vi "Periodic Tasks.vi"(8 "error in":errorcluster) -> ()   [LabVIEW 2015]
doc: "This VI runs in parallel to other tasks. It can contain as many user-defined periodic loops as you need. These can carry out PID or other sorts of timed response."
uses:
  <vilib>/Rock Robotics/WPI/Solenoid/WPI_SolenoidValue.ctl
  <vilib>/Rock Robotics/WPI/Solenoid/WPI_SolenoidSetEnum.vi
  Robot Global Data.vi
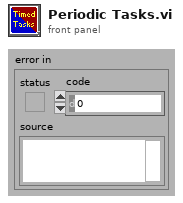
[diagram p1: front panel]
types:
  T1 = typedef "WPI_SolenoidValue.ctl" = enum16{"Off", "On", "Forward", "Reverse"}
  T2 = typedef "WPI_SolenoidDevRef.ctl" = cluster{"DevStatus":errorcluster, "Pneumatics Control Module":u8, "Forward Solenoid Channel":T3, "Reverse Solenoid Channel":T3}
  T3 = typedef "WPI_SolenoidChannel.ctl" = enum8{"Solenoid 0", "Solenoid 1", "Solenoid 2", "Solenoid 3", "Solenoid 4", "Solenoid 5", "Solenoid 6", "Solenoid 7", "Invalid"}
  T4 = typedef "WPI_MotorControlDeviceRef.ctl" = cluster{"DeviceStatus":errorcluster, "Type":T5, "PWM":cluster{"PWM Channel":T6, "DeadBand":T7}, "CAN":cluster{"Device Number":u8, "Control Mode":T8, "Semaphore":T9, "Max Vout":dbl, "TalonSRX Control Mode":T10}, "Invert":bool}
  T5 = typedef "WPI_MotorControlType.ctl" = enum16{"PWM", "CAN", "CANTalonSRX"}
  T6 = typedef "FPGA_DIOPWMChannel.ctl" = enum8{"PWM 0", "PWM 1", "PWM 2", "PWM 3", "PWM 4", "PWM 5", "PWM 6", "PWM 7", "PWM 8", "PWM 9", "PWM MXP 0", "PWM MXP 1", "PWM MXP 2", "PWM MXP 3", "PWM MXP 4", "PWM MXP 5", "PWM MXP 6", "PWM MXP 7", "PWM MXP 8", "PWM MXP 9", "Invalid"}
  T7 = typedef "WPI_PWMDeadband.ctl" = cluster{"Name":string, "maxPositivePwm":i32, "minPositivePwm":i32, "centerPwm":i32, "maxNegativePwm":i32, "minNegativePwm":i32, "angularRange":u16}
  T8 = typedef "WPI_CANJaguar_ControlMode.ctl" = enum8{"Percent VBus", "Current", "Speed", "Position", "Voltage"}
  T9 = typedef "Semaphore RefNum" = refnum<k1>
  T10 = typedef "WPI_CANTalonSRX_APIControlMode.ctl" = enum8{"Percent VBus", "Speed", "Position", "Slave", "Unchanged / Invalid", "Voltage Compensation", "Current", "Motion Profile"}
  T11 = typedef "WPI_PotentiometerDevRef.ctl" = cluster{"DevStatus":errorcluster, "Analog Channel":T12, "Invert Output":bool}
  T12 = typedef "FPGA_AIChannel.ctl" = enum8{"AI 0", "AI 1", "AI 2", "AI 3", "AI MXP 0", "AI MXP 1", "AI MXP 2", "AI MXP 3", "Invalid"}
  T13 = typedef "WPI_EncoderDevRef.ctl" = cluster{"DevStatus":errorcluster, "EncoderIndex":T14, "CounterIndex":T15, "DistancePerCount":dbl, "Decoding Type":T16}
  T14 = typedef "FPGA_EncoderIdx.ctl" = enum8{"Enc 0", "Enc 1", "Enc 2", "Enc 3", "Enc 4", "Enc 5", "Enc 6", "Enc 7", "Invalid"}
  T15 = typedef "FPGA_CounterCtrSystemIndex.ctl" = enum8{"Ctr 0", "Ctr 1", "Ctr 2", "Ctr 3", "Ctr 4", "Ctr 5", "Ctr 6", "Ctr 7", "Invalid"}
  T16 = typedef "WPI_EncoderType.ctl" = enum16{"1x", "2x", "4x"}
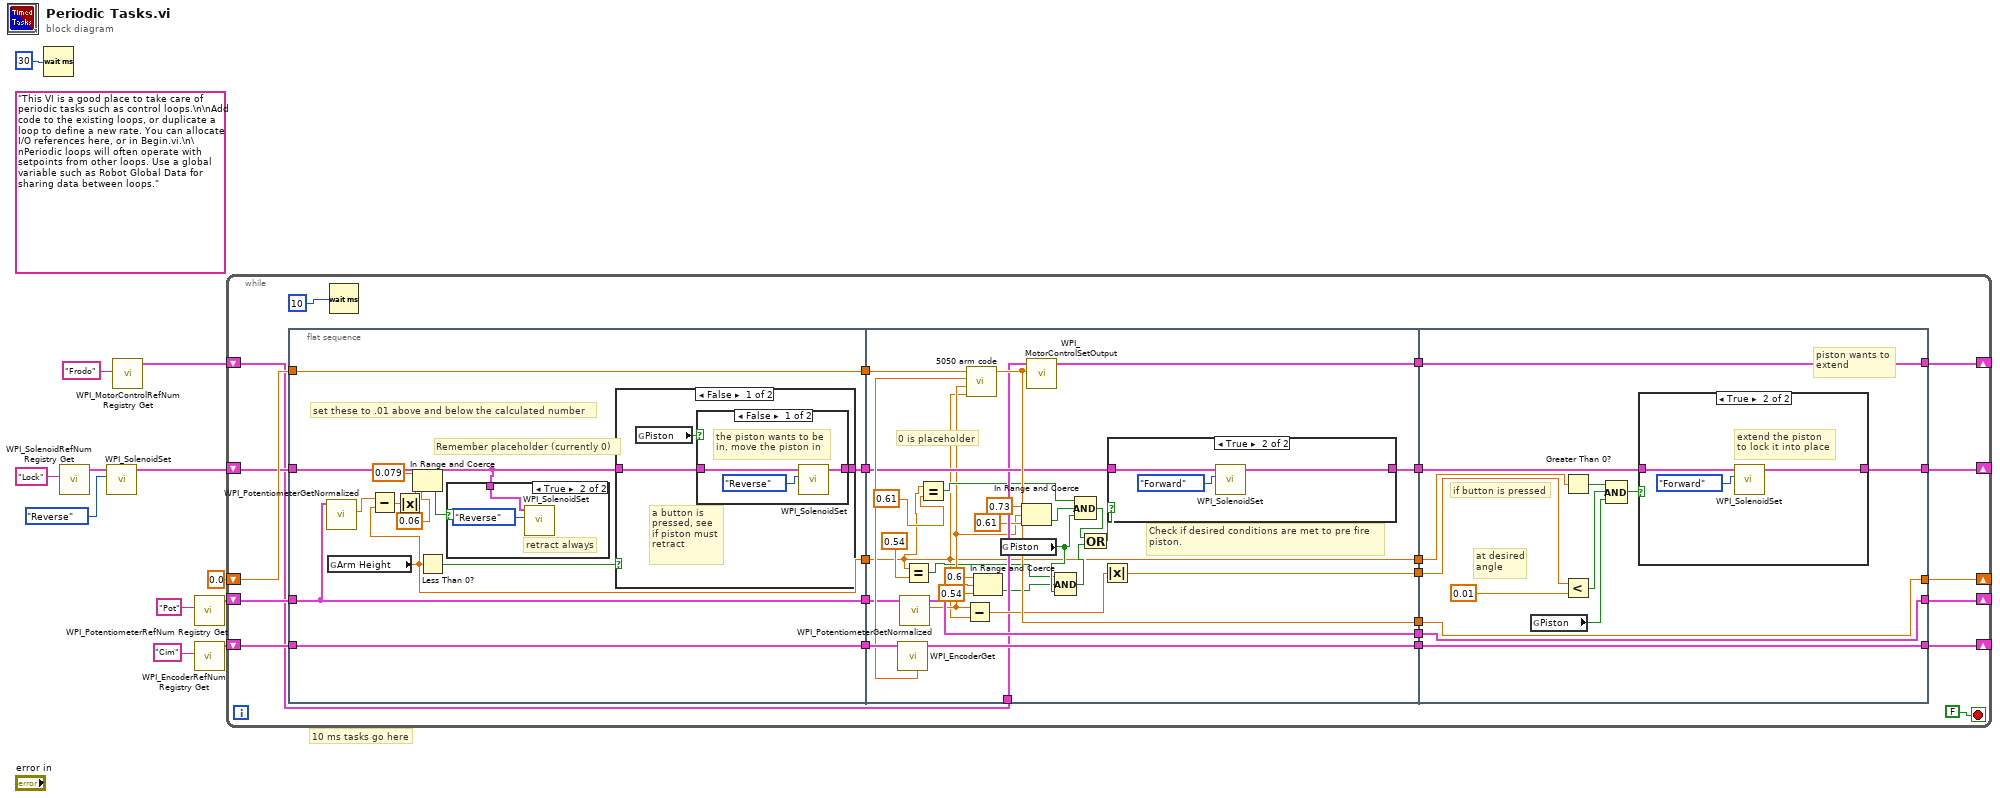
[diagram p0: block diagram]
diagram:
  (unwired) "This VI is a good place to take care of periodic tasks such as control loops.\n\nAdd code to the existing loops, or duplicate a loop to define a new rate. You can allocate I/O references here, or in Begin.vi.\n\nPeriodic loops will often operate with setpoints from other loops. Use a global variable such as Robot Global Data for sharing data between loops."
  # "10 ms tasks go here"
  n1 = Wait (ms)(milliseconds to wait=u32 30) -> ()  [unwired: 1 out]
  n2 = call <vilib>:"WPI_SolenoidRefNum Registry Get.vi"("refnum name"="Lock") -> ("SolenoidDevRef"=w4:T2)  [unwired: 9 in, 1 out]
  n3 = call-poly <vilib>:"WPI_SolenoidSet.vi"("Value"=WPI_SolenoidValue."Reverse", "SolenoidDevRef"=w4) -> ("SolenoidDevRef"=w3:T2)  [unwired: 8 in, 1 out]
  n4 = call <vilib>:"WPI_MotorControlRefNum Registry Get.vi"("refnum name"="Frodo") -> ("MotorControlDevRef"=w11:T4)  [unwired: 9 in, 1 out]
  n5 = call <vilib>:"WPI_PotentiometerRefNum Registry Get.vi"("refnum name"="Pot") -> ("PotDevRef"=w9:T11)  [unwired: 9 in, 1 out]
  n6 = call <vilib>:"WPI_EncoderRefNum Registry Get.vi"("refnum name"="Cim") -> ("EncoderDevRef"=w10:T13)  [unwired: 9 in, 1 out]
  n7 = while {
    shift-right: [w20] -> _
    shift-left: w11 -> [w14]
    shift-right: [w18] -> _
    shift-left: w9 -> [w15]
    shift-right: [w17] -> _
    shift-left: w10 -> [w22]
    shift-right: [w19] -> _
    shift-left: 0.0 -> [w24]
    shift-right: [w21] -> _
    shift-left: w3 -> [w23]
    stop <- FALSE stop-if-true
    n8 = flat-sequence {
      tunnel: w24 -> [w46]
      tunnel: w22 -> [w49]
      tunnel: [w49] -> w35
      tunnel: [w43] -> w34
      tunnel: w23 -> [w41]
      tunnel: [w47] -> w33
      tunnel: [w46] -> w32
      tunnel: [w45] -> w16
      tunnel: w15 -> [w45]
      tunnel: [w86] -> w31
      tunnel: [w85] -> w30
      tunnel: [w84] -> w29
      tunnel: [w83] -> w28
      tunnel: w35 -> [w88]
      tunnel: w34 -> [w60]
      tunnel: w33 -> [w80]
      tunnel: [w79] -> w27
      tunnel: [w60] -> w26
      tunnel: [w81] -> w25
      tunnel: w32 -> [w78]
      tunnel: w16 -> [w77]
      tunnel: w14 -> [w76]
      tunnel: [w102] -> w19
      tunnel: [w103] -> w18
      tunnel: [w104] -> w17
      tunnel: [w105] -> w20
      tunnel: w31 -> [w105]
      tunnel: w30 -> [w104]
      tunnel: w29 -> [w103]
      tunnel: w28 -> [w102]
      tunnel: w27 -> [w95]
      tunnel: w26 -> [w101]
      tunnel: w25 -> [w100]
      tunnel: [w94] -> w21
      frame #0 {
        # "set these to .01 above and below the calculated number"
        # "Remember placeholder (currently 0)"
        n9 = call <vilib>:"WPI_PotentiometerGetNormalized.vi"("PotDevRef"=w45) -> ("Normalized Value"=w44:dbl)  [unwired: 8 in, 2 out]
        n10 = global read "Robot Global Data.vi" "Arm Height"() -> (w43:dbl)
        n11 = Subtract(x=w44, y=w43) -> (x-y=w42:dbl)
        n12 = Absolute Value(x=w42) -> (abs(x)=w40:dbl)
        n13 = In Range and Coerce(upper limit=0.079, x=w40, lower limit=0.06 ("y")) -> (In Range?=w37:bool)  [unwired: 1 out]
        n14 = Less Than 0?(x=w43) -> (x < 0?=w48:bool)
        n15 = case shown="True" w37 {
          tunnel: w41 -> [_ w50]
          frame False {
            # "do nothing?"
          }
          frame True {
            # "retract always"
            n16 = call-poly <vilib>:"WPI_SolenoidSet.vi"("Value"=WPI_SolenoidValue."Reverse", "SolenoidDevRef"=w50) -> ()  [unwired: 8 in, 2 out]
          }
        }
        n17 = case shown="False" w48 {
          tunnel: w41 -> [w53 w59]
          tunnel: [w54 w59] -> w47
          frame False {
            # "a button is\npressed, see\nif piston must\nretract"
            n18 = global read "Robot Global Data.vi" "Piston"() -> (w52:bool)
            n19 = case shown="False" w52 {
              tunnel: [w55 w58] -> w54
              tunnel: w53 -> [w57 w58]
              frame False {
                # "the piston wants to be\nin, move the piston in"
                n20 = call-poly <vilib>:"WPI_SolenoidSet.vi"("Value"=WPI_SolenoidValue."Reverse", "SolenoidDevRef"=w57) -> ("SolenoidDevRef"=w55:T2)  [unwired: 8 in, 1 out]
              }
              frame True {
                # "the piston wants to\nbe out, do not extend\npiston yet"
              }
            }
          }
          frame True {
            # "no button is pressed\ndo not change piston position"
          }
        }
      }
      frame #1 {
        # "0 is placeholder"
        # "Check if desired conditions are met to pre fire piston."
        n21 = call <vilib>:"WPI_EncoderGet.vi"("EncoderDevRef"=w88) -> ("EncoderDevRef"=w85:T13, "Rate"=w87:dbl)  [unwired: 5 in, 4 out]
        n22 = call <vilib>:"WPI_PotentiometerGetNormalized.vi"("PotDevRef"=w77) -> ("Normalized Value"=w65:dbl, "PotDevRef"=w84:T11)  [unwired: 8 in, 1 out]
        n23 = Equal?(x=w60, y=0.54) -> (x = y?=w62:bool)
        n24 = Equal?(x=w60, y=0.61 ("value")) -> (x = y?=w71:bool)
        n25 = Subtract(x=w65, y=w60) -> (x-y=w82:dbl)
        n26 = call "5050 arm code.vi"("desiredAngle"=w60, "potAngle"=w65, "encoderHz"=w87, "initSpeed"=w78) -> ("motorSpeed"=w83:dbl)  [unwired: 7 in]
        n27 = In Range and Coerce(upper limit=0.6, x=w65, lower limit=0.54) -> (In Range?=w66:bool)  [unwired: 1 out]
        n28 = global read "Robot Global Data.vi" "Piston"() -> (w67:bool)
        n29 = In Range and Coerce(upper limit=0.73, x=w65, lower limit=0.61) -> (In Range?=w72:bool)  [unwired: 1 out]
        n30 = call <vilib>:"WPI_MotorControlSetOutput.vi"("Output"=w83, "MotorControlDevRef"=w76) -> ("MotorControlDevRef"=w86:T4)  [unwired: 7 in, 2 out]
        n31 = Compound Arithmetic op=AND(w62, w66, w67) -> (w68:bool)
        n32 = Compound Arithmetic op=AND(w71, w72, w67) -> (w70:bool)
        n33 = Compound Arithmetic op=OR(w70, w68) -> (w69:bool)
        n34 = Absolute Value(x=w82) -> (abs(x)=w81:dbl)
        n35 = case shown="True" w69 {
          tunnel: w80 -> [w89 w91]
          tunnel: [w89 w90] -> w79
          frame False {
          }
          frame True {
            n36 = call-poly <vilib>:"WPI_SolenoidSet.vi"("Value"=WPI_SolenoidValue."Forward", "SolenoidDevRef"=w91) -> ("SolenoidDevRef"=w90:T2)  [unwired: 8 in, 1 out]
          }
        }
      }
      frame #2 {
        # "piston wants to\nextend"
        # "at desired\nangle"
        # "if button is pressed"
        n37 = global read "Robot Global Data.vi" "Piston"() -> (w93:bool)
        n38 = Greater Than 0?(x=w101) -> (x > 0?=w97:bool)
        n39 = Less?(x=w100, y=0.01) -> (x < y?=w96:bool)
        n40 = Compound Arithmetic op=AND(w97, w96, w93) -> (w98:bool)
        n41 = case shown="True" w98 {
          tunnel: w95 -> [w106 w109]
          tunnel: [w106 w108] -> w94
          frame False {
            # "do not extend piston"
            # "either arm is not\nwhere it is supposed\nto be, or the piston\ndoesn't want to\nextend, or someone\nlet go of the button"
          }
          frame True {
            # "extend the piston\nto lock it into place"
            n42 = call-poly <vilib>:"WPI_SolenoidSet.vi"("Value"=WPI_SolenoidValue."Forward", "SolenoidDevRef"=w109) -> ("SolenoidDevRef"=w108:T2)  [unwired: 8 in, 1 out]
          }
        }
      }
    }
    n43 = Wait (ms)(milliseconds to wait=10) -> ()  [unwired: 1 out]
  }
